vi "Teleop.vi"(10 "Match Info":T1={"Autonomous Elapsed Seconds"=0.0, "TeleOp Elapsed Seconds"=0.0, "Disabled Elapsed Seconds"=0.0, "Visited Autonomous"=FALSE, "Visited TeleOp"=FALSE, "Visited Disabled"=FALSE, "Autonomous Settings"={"Autonomous Style"=enum."Independent", "VI Refnum"=refnum}}, 11 "Call Context":T2) -> ()   [LabVIEW 2014]
doc: "This VI is called for each TeleOp packet received from the DS where the robot is not disabled. It is often used to read from the joysticks and update I/O or to update setpoints for timed control loops. It should complete and return within 20 milliseconds or it may miss DS packets."
uses:
  <vilib>/Rock Robotics/WPI/DriverStation/WPI_DriverStationDerivedRobotMode.ctl
  <vilib>/Rock Robotics/WPI/DriverStation/WPI_DriverStationMatch Info.ctl
  <vilib>/Rock Robotics/WPI/Joystick/WPI_JoystickGetSetRefNum.vi
  <vilib>/Rock Robotics/WPI/RobotDrive/WPI_RobotDriveGetSetRefNum.vi
  <vilib>/Rock Robotics/Network Tables/SD Read Boolean.vi
  Robot Global Data.vi
  <vilib>/Rock Robotics/Network Tables/SD Write Boolean Array.vi
  <vilib>/Rock Robotics/Network Tables/SD Write Numeric Array.vi
  <vilib>/Rock Robotics/WPI/RobotDrive/WPI_RobotDriveMecanumDrive_Cartesian.vi
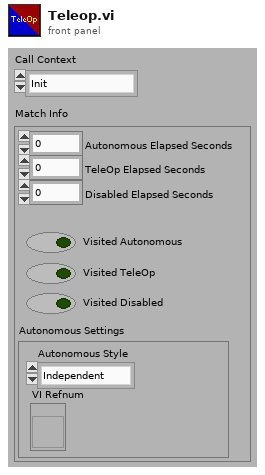
[diagram p1: front panel]
types:
  T1 = typedef "WPI_DriverStationMatch Info.ctl" = cluster{"Autonomous Elapsed Seconds":dbl, "TeleOp Elapsed Seconds":dbl, "Disabled Elapsed Seconds":dbl, "Visited Autonomous":bool, "Visited TeleOp":bool, "Visited Disabled":bool, "Autonomous Settings":cluster{"Autonomous Style":enum16{"Iterative", "Independent"}, "VI Refnum":refnum<vi>}}
  T2 = typedef "WPI_DriverStationDerivedRobotMode.ctl" = enum16{"Init", "Execute", "Stop"}
  T3 = typedef "WPI_JoystickDevRef.ctl" = cluster{"Device":T4}
  T4 = typedef "WPI_JoystickDeviceEnum.ctl" = enum16{"USB 0", "USB 1", "USB 2", "USB 3", "USB 4", "USB 5"}
  T5 = typedef "WPI_RobotDriveDevRef.ctl" = cluster{"DevStatus":errorcluster, "Motors[]":T6[], "Square Inputs":bool, "Max Output":dbl}
  T6 = typedef "WPI_MotorControlDeviceRef.ctl" = cluster{"DeviceStatus":errorcluster, "Type":T7, "PWM":cluster{"Controller":T8, "PWM Channel":T9, "DeadBand":T10}, "CAN":cluster{"Device Number":u8, "Control Mode":T11, "Semaphore":T12, "Max Vout":dbl, "TalonSRX Control Mode":T13}, "Invert":bool, "TransformRef":T14, "InvTransformRef":T14}
  T7 = typedef "WPI_MotorControlType.ctl" = enum16{"PWM", "CAN", "CANTalonSRX"}
  T8 = typedef "FPGA_TypedefDigitalModule.ctl" = enum16{"Controller 1"}
  T9 = typedef "FPGA_DIOPWMChannel.ctl" = enum8{"PWM 0", "PWM 1", "PWM 2", "PWM 3", "PWM 4", "PWM 5", "PWM 6", "PWM 7", "PWM 8", "PWM 9", "PWM MXP 0", "PWM MXP 1", "PWM MXP 2", "PWM MXP 3", "PWM MXP 4", "PWM MXP 5", "PWM MXP 6", "PWM MXP 7", "PWM MXP 8", "PWM MXP 9", "Invalid"}
  T10 = typedef "WPI_PWMDeadband.ctl" = cluster{"Name":string, "maxPositivePwm":i32, "minPositivePwm":i32, "centerPwm":i32, "maxNegativePwm":i32, "minNegativePwm":i32, "angularRange":u16}
  T11 = typedef "WPI_CANJaguar_ControlMode.ctl" = enum8{"Percent VBus", "Current", "Speed", "Position", "Voltage"}
  T12 = typedef "Semaphore RefNum" = refnum<k1>
  T13 = typedef "WPI_CANTalonSRX_APIControlMode.ctl" = enum8{"Percent VBus", "Speed", "Position", "Slave", "Unchanged / Invalid"}
  T14 = typedef "WPI_PWMTransform_ConPane.ctl" = refnum<vi>
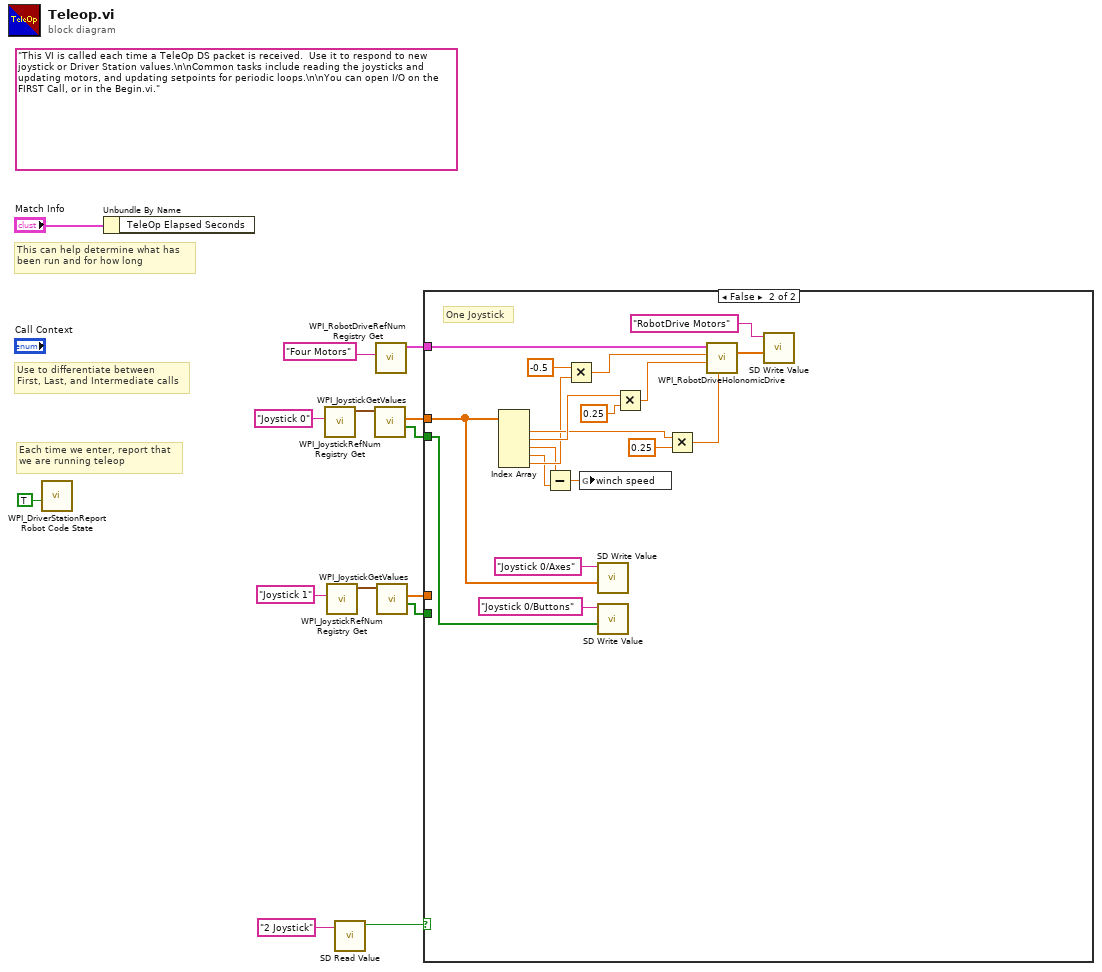
[diagram p0: block diagram]
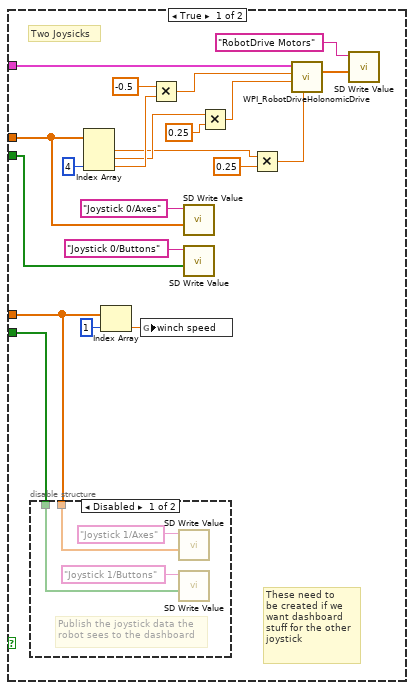
[diagram p2: hidden frame]
diagram:
  (unwired) "This VI is called each time a TeleOp DS packet is received.  Use it to respond to new joystick or Driver Station values.\n\nCommon tasks include reading the joysticks and updating motors, and updating setpoints for periodic loops.\n\nYou can open I/O on the FIRST Call, or in the Begin.vi."
  # "Each time we enter, report that\nwe are running teleop"
  # "Use to differentiate between\nFirst, Last, and Intermediate calls"
  # "This can help determine what has\nbeen run and for how long"
  n1 = call <vilib>:"WPI_DriverStationReport Robot Code State.vi"("TeleOp"=TRUE ("Autonomous")) -> ()  [unwired: 10 in, 1 out]
  n2 = Unbundle By Name("Match Info") -> ()  [unwired: 1 out]
  n3 = call <vilib>:"WPI_JoystickRefNum Registry Get.vi"("refnum name"="Joystick 0") -> ("JoystickDevRef"=w10:T3)  [unwired: 1 in, 9 out]
  n4 = call <vilib>:"WPI_JoystickRefNum Registry Get.vi"("refnum name"="Joystick 1") -> ("JoystickDevRef"=w11:T3)  [unwired: 1 in, 9 out]
  n5 = call-poly <vilib>:"SD Read Value.vi"("Name"="2 Joystick") -> ("Boolean"=w2:bool)  [unwired: 8 in, 2 out]
  n6 = call <vilib>:"WPI_JoystickGetValues.vi"("JoystickDevRef"=w10) -> ("Buttons"=w5:bool[], "Axes"=w6:dbl[])  [unwired: 6 in, 3 out]
  n7 = call <vilib>:"WPI_RobotDriveRefNum Registry Get.vi"("refnum name"="Four Motors") -> ("RobotDriveDevRef"=w7:T5)  [unwired: 1 in, 9 out]
  n8 = call <vilib>:"WPI_JoystickGetValues.vi"("JoystickDevRef"=w11) -> ("Buttons"=w3:bool[], "Axes"=w4:dbl[])  [unwired: 6 in, 3 out]
  n9 = case shown="False" w2 {
    tunnel: w7 -> [w23 w48]
    tunnel: w6 -> [w19 w45]
    tunnel: w5 -> [w20 w43]
    tunnel: w4 -> [w15 _]
    tunnel: w3 -> [w16 _]
    frame True {
      # "Two Joysicks"
      # "These need to\nbe created if we\nwant dashboard\nstuff for the other\njoystick"
      n10 = disable-structure shown="Disabled" {
        disable-tunnel: w16 -> [w39 _]
        disable-tunnel: w15 -> [w38 _]
        frame Disabled {
          # "Publish the joystick data the\nrobot sees to the dashboard"
          n11 = call-poly <vilib>:"SD Write Value.vi"("Numeric Array"=w38, "Name"="Joystick 1/Axes") -> ()  [unwired: 8 in, 2 out]
          n12 = call-poly <vilib>:"SD Write Value.vi"("Boolean Array"=w39, "Name"="Joystick 1/Buttons") -> ()  [unwired: 8 in, 2 out]
        }
        frame Enabled {
        }
      }
      n13 = Index Array(array=w19, index #3=4 ("index")) -> (element #1=w29:dbl, element #2=w31:dbl, element #3=w35:dbl)  [unwired: 2 in]
      n14 = Index Array(array=w15, index=1) -> (element=w17:dbl)
      n15 = global write "Robot Global Data.vi" "winch speed"(w17) -> ()
      n16 = Multiply(x=-0.5, y=w35) -> (x*y=w26:dbl)
      n17 = call-poly <vilib>:"SD Write Value.vi"("Numeric Array"=w19, "Name"="Joystick 0/Axes") -> ()  [unwired: 8 in, 2 out]
      n18 = call-poly <vilib>:"SD Write Value.vi"("Boolean Array"=w20, "Name"="Joystick 0/Buttons") -> ()  [unwired: 8 in, 2 out]
      n19 = Multiply(x=w31, y=0.25) -> (x*y=w28:dbl)
      n20 = Multiply(x=w29, y=0.25) -> (x*y=w27:dbl)
      n21 = call-poly <vilib>:"WPI_RobotDriveHolonomicDrive.vi"("Rotation"=w27, "y"=w28, "X"=w26, "RobotDriveDevRef"=w23) -> ("Motor Values"=w25:dbl[])  [unwired: 5 in, 2 out]
      n22 = call-poly <vilib>:"SD Write Value.vi"("Numeric Array"=w25, "Name"="RobotDrive Motors") -> ()  [unwired: 8 in, 2 out]
    }
    frame False {
      # "One Joystick"
      n23 = Index Array(array=w45) -> (element #1=w54:dbl, element #2=w56:dbl, element #3=w40:dbl, element #4=w41:dbl, element #5=w44:dbl)  [unwired: 5 in]
      n24 = Subtract(x=w40, y=w41) -> (x-y=w42:dbl)
      n25 = Multiply(x=-0.5, y=w44) -> (x*y=w51:dbl)
      n26 = global write "Robot Global Data.vi" "winch speed"(w42) -> ()
      n27 = call-poly <vilib>:"SD Write Value.vi"("Numeric Array"=w45, "Name"="Joystick 0/Axes") -> ()  [unwired: 8 in, 2 out]
      n28 = call-poly <vilib>:"SD Write Value.vi"("Boolean Array"=w43, "Name"="Joystick 0/Buttons") -> ()  [unwired: 8 in, 2 out]
      n29 = Multiply(x=w56, y=0.25) -> (x*y=w53:dbl)
      n30 = Multiply(x=w54, y=0.25) -> (x*y=w52:dbl)
      n31 = call-poly <vilib>:"WPI_RobotDriveHolonomicDrive.vi"("Rotation"=w52, "y"=w53, "X"=w51, "RobotDriveDevRef"=w48) -> ("Motor Values"=w50:dbl[])  [unwired: 5 in, 2 out]
      n32 = call-poly <vilib>:"SD Write Value.vi"("Numeric Array"=w50, "Name"="RobotDrive Motors") -> ()  [unwired: 8 in, 2 out]
    }
  }
